vi "HP34970A List to Array.vi"(4 "List (empty)":string, 7 "Separator (,)":string=",") -> (0 "Output Number Array":dbl[](array[numeric]) format="%.2f", 3 "Output String Array":string[](array[string]))   [LabVIEW 2020]
doc: "Given a List of strings separated by a Separator, this VI returns the List as a String Array. If the strings are numbers, a Number Array is also returned."
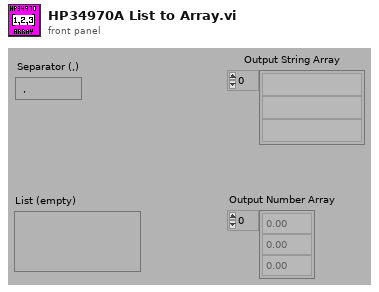
[diagram p1: front panel]
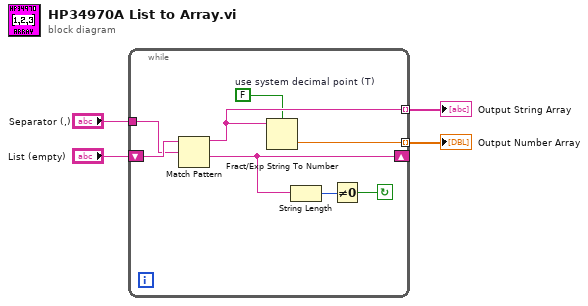
[diagram p0: block diagram]
diagram:
  n1 = while {
    shift-right: [w8] -> _
    shift-left: "List (empty)" -> [w10]
    tunnel: [w9] -> w3 mode=indexing
    tunnel: [w7] -> w2 mode=indexing
    tunnel: "Separator (,)" -> [w6]
    stop <- w12 continue-if-true
    w5 = FALSE  # use system decimal point (T)
    n2 = Match Pattern(string=w10, regular expression=w6) -> (before substring=w7:string, after substring=w8:string)  [unwired: 1 in, 2 out]
    n3 = Fract/Exp String To Number(use system decimal point (T)=w5, string=w7) -> (number=w9:dbl)  [unwired: 2 in, 1 out]
    n4 = String Length(string=w8) -> (length=w11:i32)
    n5 = Not Equal To 0?(x=w11) -> (x != 0?=w12:bool)
  }
  "Output Number Array" <- w3
  "Output String Array" <- w2
